vi "LWXPS_PositionerSGammaPreviousMotionTimesGet.vi"(8 "LabVIEW error IN":errorcluster, 10 "Positioner Name":string, 11 "XPS Reference IN":refnum<k24>) -> (0 "XPS Error String":string, 1 "Settling time":dbl, 2 "Setting time":dbl, 3 "Returned error code":i32, 4 "LabVIEW error OUT":errorcluster, 5 "XPS Reference OUT":refnum<k24>)   [LabVIEW 2014]
uses:
  D:/XPSQ8_LabView_Library/Development/Source/Dll/Newport.XPS.CommandInterface.dll
  Dll/Newport.XPS.CommandInterface.dll
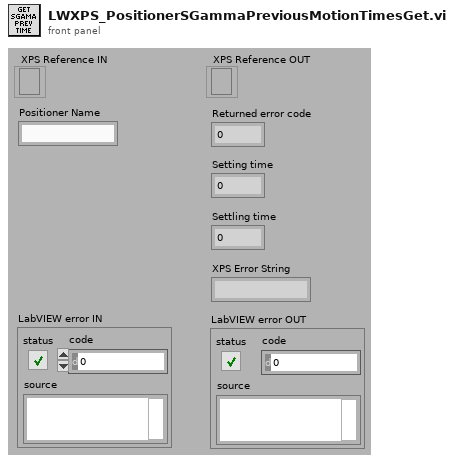
[diagram p1: front panel]
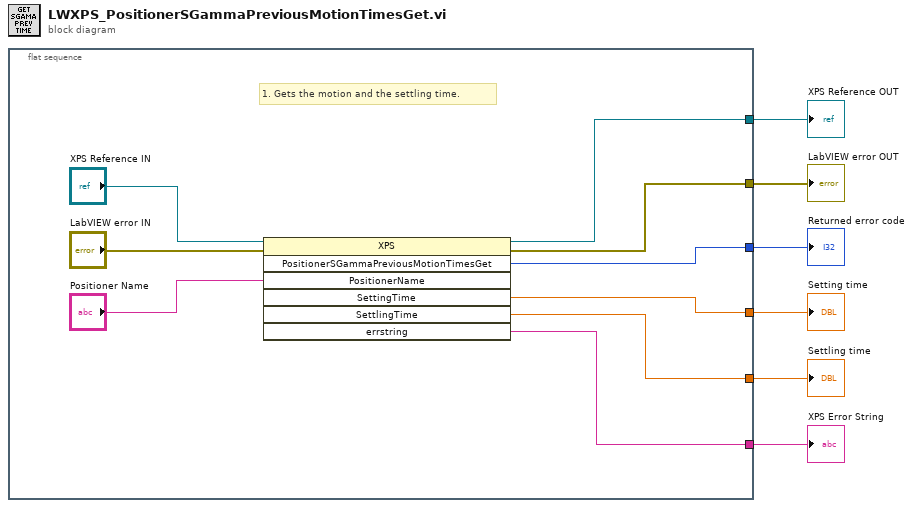
[diagram p0: block diagram]
diagram:
  n1 = flat-sequence {
    tunnel: [w13] -> w6
    tunnel: [w10] -> w5
    tunnel: [w14] -> w4
    tunnel: [w8] -> w2
    tunnel: [w9] -> w3
    tunnel: [w7] -> w1
    frame #0 {
      # "1. Gets the motion and the settling time."
      n2 = invoke class="XPS" method="PositionerSGammaPreviousMotionTimesGet"(reference="XPS Reference IN", error in="LabVIEW error IN", "PositionerName"="Positioner Name") -> (reference out=w13:refnum<k24>, error out=w10:errorcluster, "PositionerSGammaPreviousMotionTimesGet"=w14:i32, "SettingTime"=w8:dbl, "SettlingTime"=w9:dbl, "errstring"=w7:string)  [unwired: 4 in, 1 out]
    }
  }
  "XPS Error String" <- w1
  "XPS Reference OUT" <- w6
  "LabVIEW error OUT" <- w5
  "Returned error code" <- w4
  "Settling time" <- w3
  "Setting time" <- w2
